vi "subDAQ_SetPatchAO.vi"(6 "DAQ ports":T1={"Lasers DO lines"=["Dev2/port0/line0", "Dev2/port0/line1", "Dev2/port0/line2", "Dev2/port0/line3", "Dev2/port0/line4", "Dev2/port0/line5"], "Lasers AO lines"=["Dev2/ao0", "Dev2/ao1", "Dev2/ao2", "Dev2/ao3", "Dev2/ao4", "Dev2/ao5"], "Patch AO line"="Dev1/ao1", "Patch AI lines 1"={"Patch scaled output"="Dev1/ai8", "Patch 10 V_m "="Dev1/ai0"}, "Camera timing DI"="Dev1/port0/line8", "Dev1 timing DO "="Dev1/port0/line9", "Dev1 trigger source"="/Dev1/PFI0", "Dev2 trigger source"="/Dev2/PFI0", "LED line"="Dev1/port0/line0", "Global Shutter line"="Dev2/port0/line6", "Patch AI lines 2"={"Cell capacitance"="Dev1/ai1", "Mode"="Dev1/ai2", "Frequency"="Dev1/ai3", "Gain"="Dev1/ai4"}}, 7 "Patch Ex. Command AO signal (0V)":dbl format="%0.2f", 8 "Error in (no error)":errorcluster) -> (0 "Error out":errorcluster)   [LabVIEW 2015]
panel:
  # "637"
  # "561"
  # "532"
  # "488"
  # "405"
  # "Red"
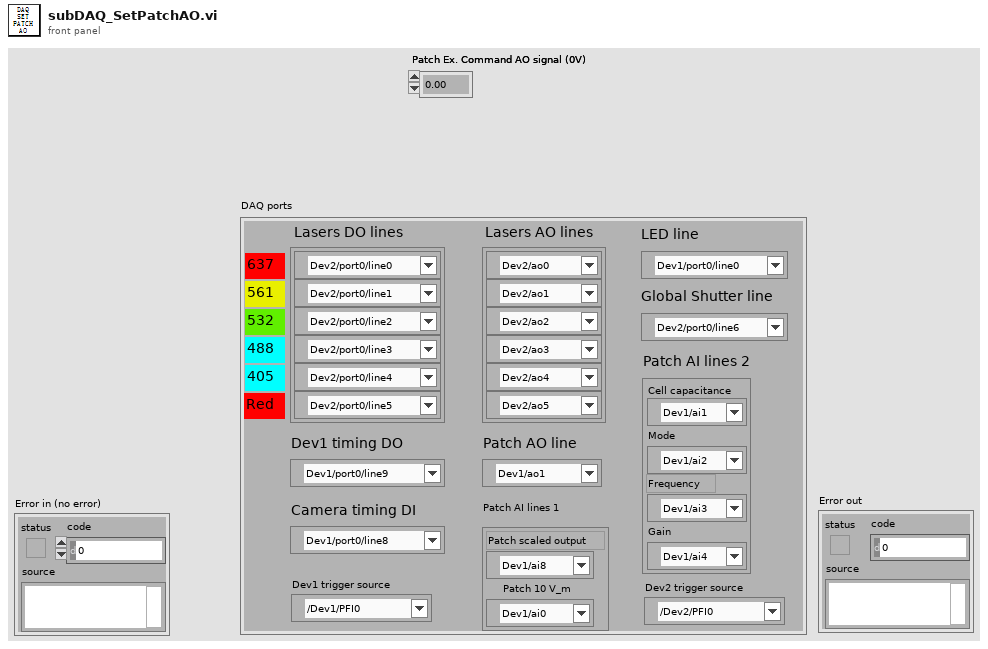
[diagram p1: front panel]
types:
  T1 = cluster{"Lasers DO lines":tag[], "Lasers AO lines":tag[], "Patch AO line":tag, "Patch AI lines 1":cluster{"Patch scaled output":tag, "Patch 10 V_m ":tag}, "Camera timing DI":tag, "Dev1 timing DO ":tag, "Dev1 trigger source":tag, "Dev2 trigger source":tag, "LED line":tag, "Global Shutter line":tag, "Patch AI lines 2":cluster{"Cell capacitance":tag, "Mode":tag, "Frequency":tag, "Gain":tag}}
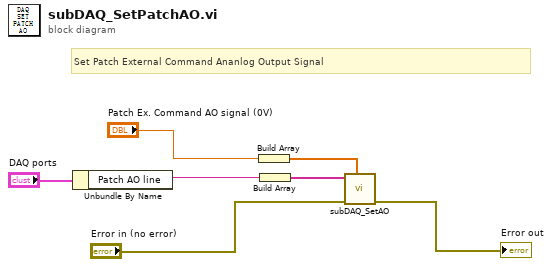
[diagram p0: block diagram]
diagram:
  # "Set Patch External Command Ananlog Output Signal"
  n1 = Unbundle By Name("DAQ ports") -> ("Patch AO line"=w6:tag)
  n2 = Build Array("Patch Ex. Command AO signal (0V)") -> (w4:dbl[])
  n3 = Build Array(w6) -> (w3:tag[])
  n4 = call "subDAQ_SetAO.vi"("Analog value array"=w4, "error in (no error)"="Error in (no error)", "Analog line array"=w3) -> ("error out"=→"Error out":errorcluster)  [unwired: 8 in]
